vi "dfd_FXP PtByPt Lattice AR (normalized).vi"(6 "state in":i64[](array[numeric]), 7 "FXPOPs":T5[](array[typedef]) {"source" items=["Coef a/k"=0, "Coef b/v"=7, "Input"=1, "Output"=2, "Multiplicand"=3, "Product"=4, "Sum"=5, "Delay"=6, "Gain"=8]}, 8 "filtering statistics in":T3(array[cluster]) {"statistics information"."min value" format="%.2f"; "statistics information"."max value" format="%.2f"; "Quantizer Source" items=["Coefficients a/k"=0, "Coefficients b/v"=7, "Input"=1, "Output"=2, "Multiplicand"=3, "Product"=4, "Sum"=5, "Delay"=6]}, 9 "coef ^k[M..1]":T4, 10 "coef k[M..1]":T4, 11 "x":T7={"value"=0, "wl"=0, "iwl"=0, "Signed"=TRUE} {"value" format="%.0x"}) -> (0 "filtering statistics out":T3(array[cluster]) {"statistics information"."min value" format="%.2f"; "statistics information"."max value" format="%.2f"; "Quantizer Source" items=["Coefficients a/k"=0, "Coefficients b/v"=7, "Input"=1, "Output"=2, "Multiplicand"=3, "Product"=4, "Sum"=5, "Delay"=6]}, 3 "filtered x":T7={"value"=0, "wl"=0, "iwl"=0, "Signed"=TRUE} {"value" format="%.0x"}, 4 "state out":i64[](array[numeric]))   [LabVIEW 2017, in "NI_DigFilter_FXP.lvlib"]
uses:
  <vilib>/addons/Digital Filter Design/NI_DigFilter_FXP.lvlib
  <vilib>/addons/Digital Filter Design/_Objects.llb/dfd_DFXP Data Type (scaler).ctl
  <vilib>/addons/Digital Filter Design/_Objects.llb/dfd_DFXP Operation Parameter.ctl
  <vilib>/addons/Digital Filter Design/_Objects.llb/dfd_Internal Quantization Srcs.ctl
  <vilib>/addons/Digital Filter Design/_Objects.llb/dfd_DFXP Data Type (vector).ctl
  <vilib>/addons/Digital Filter Design/_Objects.llb/DFD Quantization Sources.ctl
  <vilib>/addons/Digital Filter Design/_Objects.llb/DFD FXP Statistics Data.ctl
  <vilib>/addons/Digital Filter Design/NI_DigFilterLicensed.lvlib
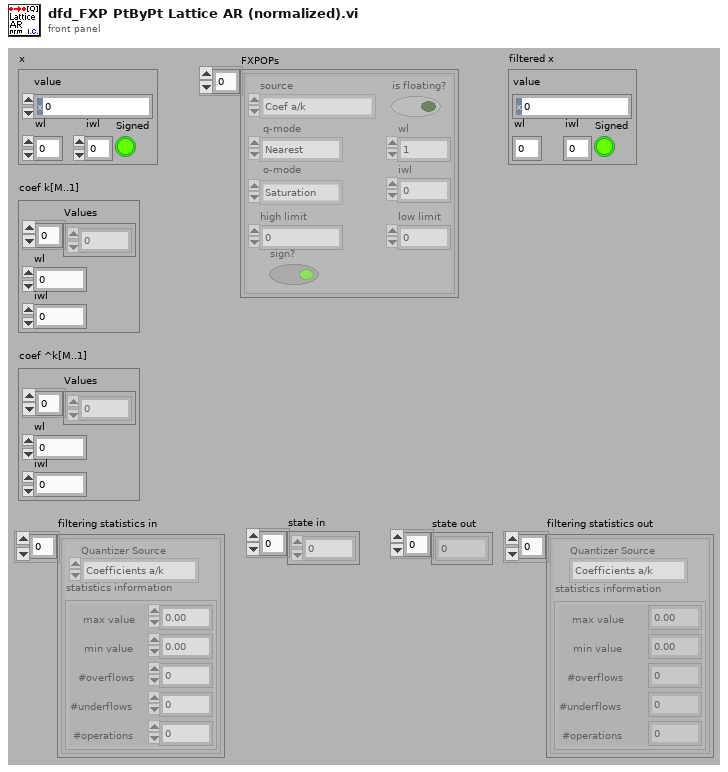
[diagram p1: front panel]
types:
  T1 = typedef "NI_DigFilterLicensed.lvlib/DFD Quantization Sources.ctl" = u16
  T2 = typedef "NI_DigFilterLicensed.lvlib/DFD FXP Statistics Data.ctl" = cluster{"max value":ext, "min value":ext, "#overflows":i32, "#underflows":i32, "#operations":i32}
  T3 = cluster{"Quantizer Source":T1, "statistics information":T2}[]
  T4 = typedef "dfd_DFXP Data Type (vector).ctl" = cluster{"Values":i64[], "wl":i16, "iwl":i16}
  T5 = typedef "dfd_DFXP Operation Parameter.ctl" = cluster{"source":T6, "is floating?":bool, "o-mode":enum16{"Saturation", "Wrap"}, "q-mode":enum16{"Nearest", "Truncation"}, "wl":i16, "high limit":i64, "low limit":i64, "iwl":i16, "sign?":bool}
  T6 = typedef "NI_DigFilterLicensed.lvlib/dfd_Internal Quantization Srcs.ctl" = u16
  T7 = typedef "dfd_DFXP Data Type (scaler).ctl" = cluster{"value":i64, "wl":i16, "iwl":i16, "Signed":bool}
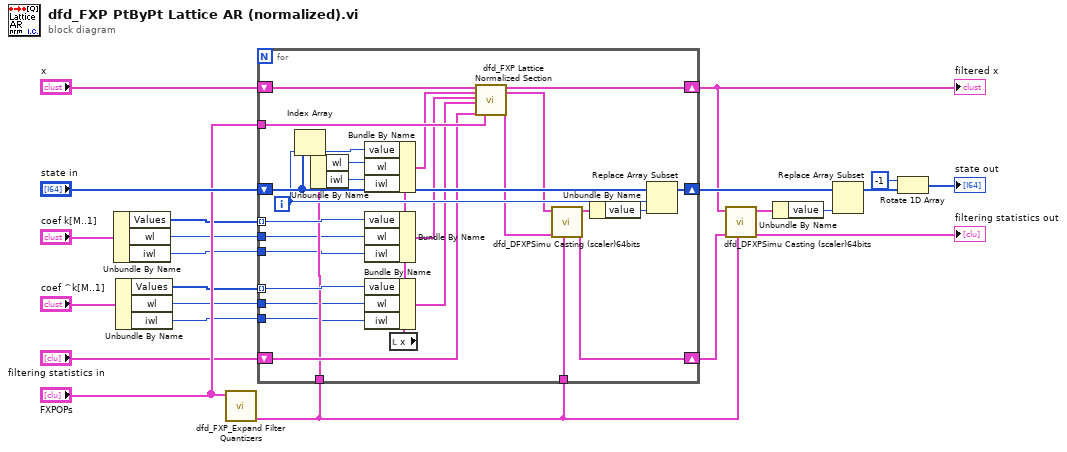
[diagram p0: block diagram]
diagram:
  n1 = Unbundle By Name("coef k[M..1]") -> ("Values"=w8:i64[], "wl"=w5:i16, "iwl"=w4:i16)
  n2 = Unbundle By Name("coef ^k[M..1]") -> ("Values"=w7:i64[], "wl"=w3:i16, "iwl"=w2:i16)
  n3 = call <vilib>:"dfd_FXP_Expand Filter Quantizers.vi"("FXPOPs"="FXPOPs") -> ("Delay"=w6:T5)  [unwired: 10 out]
  n4 = for {
    shift-right: [w42] -> w16
    shift-left: "x" -> [w45]
    shift-right: [w48] -> w19
    shift-left: "state in" -> [w49]
    tunnel: w6 -> [w37]
    tunnel: "FXPOPs" -> [w41]
    shift-right: [w38] -> w12
    shift-left: "filtering statistics in" -> [w40]
    tunnel: w8 -> [w36] mode=indexing
    tunnel: w7 -> [w35] mode=indexing
    tunnel: w6 -> [w33]
    tunnel: w5 -> [w29]
    tunnel: w4 -> [w28]
    tunnel: w3 -> [w25]
    tunnel: w2 -> [w24]
    i -> [w46]
    n5 = Index Array(array=w49, index=w46) -> (element=w44:i64)
    n6 = Unbundle By Name(w33) -> ("wl"=w32:i16, "iwl"=w31:i16)
    n7 = local read "x"() -> (w26:T7)
    n8 = Bundle By Name(cluster=w26, "value"=w44, "wl"=w32, "iwl"=w31) -> (w34:T7)
    n9 = Bundle By Name(cluster=w26, "value"=w36, "wl"=w29, "iwl"=w28) -> (w30:T7)
    n10 = Bundle By Name(cluster=w26, "value"=w35, "wl"=w25, "iwl"=w24) -> (w27:T7)
    n11 = call <vilib>:"dfd_FXP Lattice Normalized Section.vi"("x(m)"=w45, "w(m-1)"=w34, "k(m)"=w30, "^k(m)"=w27, "filtering statistics in"=w40, "FXPOPs"=w41) -> ("x(m-1)"=w42:T7, "w(m)"=w43:T7, "filtering statistics out"=w39:T3)  [unwired: 11 out]
    n12 = call <vilib>:"dfd_DFXPSimu Casting (scaler)64bits.vi"("op params"=w37, "filtering statistics in"=w39, "Value in"=w43) -> ("filtering statistics out"=w38:T3, "Value out"=w47:T7)  [unwired: 2 in, 5 out]
    n13 = Unbundle By Name(w47) -> ("value"=w23:i64)
    n14 = Replace Array Subset(array=w49, new element=w23, index=w46) -> (w48:i64[])
  }
  "filtered x" <- w16
  n15 = call <vilib>:"dfd_DFXPSimu Casting (scaler)64bits.vi"("op params"=w6, "filtering statistics in"=w12, "Value in"=w16) -> ("filtering statistics out"=→"filtering statistics out":T3, "Value out"=w18:T7)  [unwired: 2 in, 5 out]
  n16 = Unbundle By Name(w18) -> ("value"=w1:i64)
  n17 = Replace Array Subset(array=w19, new element=w1) -> (w14:i64[])  [unwired: 1 in]
  n18 = Rotate 1D Array(1:w14, 2:-1 ("n")) -> (0:→"state out":i64[])
